vi "GetBin16.vi"(8 "error in (no error)":errorcluster, 11 "MsgPackDeserializer in":refnum<class "MsgPackDeserializer.lvclass">) -> (0 "error out":errorcluster, 2 "data":string, 3 "MsgPackDeserializer out":refnum<class "MsgPackDeserializer.lvclass">)   [LabVIEW 2015, in "MsgPackDeserializer.lvclass"]
uses:
  MsgPackDeserializer.lvclass
  MsgPackDeserializer.lvclass/MsgPackDeserializer.ctl
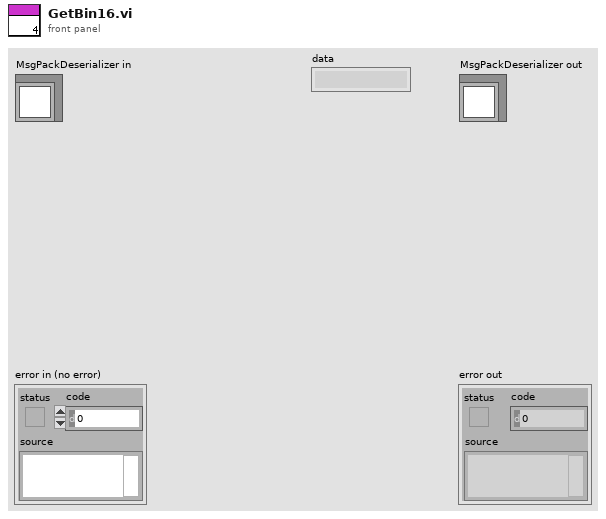
[diagram p1: front panel]
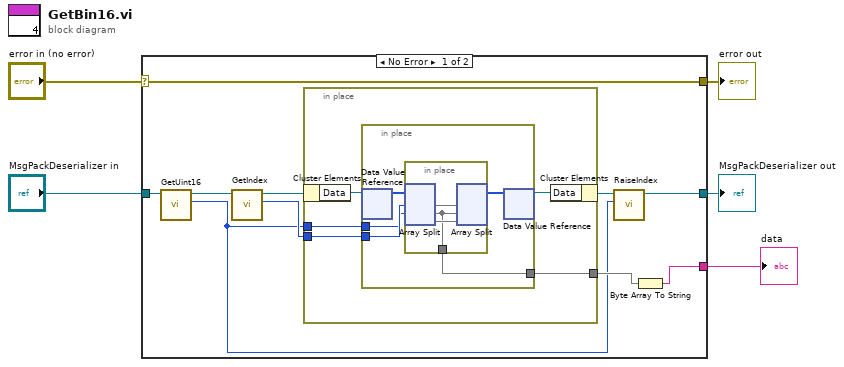
[diagram p0: block diagram]
diagram:
  n1 = case shown="No Error" "error in (no error)" {
    selector: "error in (no error)" -> [w15 w30]
    tunnel: [w15 w30] -> w4
    tunnel: [w7 w29] -> w2
    tunnel: "MsgPackDeserializer in" -> [w11 w29]
    tunnel: [w6 _] -> w1
    frame No Error {
      n2 = call "GetUint16.vi"("MsgPackDeserializer in"=w11) -> ("Number"=w8:u16, "MsgPackDeserializer out"=w10:refnum<class "MsgPackDeserializer.lvclass">)  [unwired: 8 in, 1 out]
      n3 = call "GetIndex.vi"("MsgPackDeserializer in"=w10) -> ("Index"=w12:i64, "MsgPackDeserializer out"=w13:refnum<class "MsgPackDeserializer.lvclass">)  [unwired: 8 in, 1 out]
      n4 = in-place {
        in-place-border: w12 -> [w18]
        in-place-border: w8 -> [w17]
        in-place-border: [w16] -> w9
        n5 = in-place-cluster #1(w13) -> ("Data"=w20:refnum<data-value>)
        n6 = in-place {
          in-place-border: w18 -> [w24]
          in-place-border: w17 -> [w23]
          in-place-border: [w22] -> w16
          n7 = in-place-dvr #2(w20) -> (w25:u8[])  [unwired: 1 out]
          n8 = in-place {
            in-place-border: [w26] -> w22
            n9 = in-place-split #3(w25, w24, w23) -> (w27:u8[], w26:u8[], w28:u8[])
            n10 = in-place-split #3(w27, w26, w28) -> (w21:u8[])  [unwired: 2 out]
          }
          n11 = in-place-dvr #2(w21) -> (w19:refnum<data-value>)  [unwired: 1 out]
        }
        n12 = in-place-cluster #1("Data"=w19) -> (w14:refnum<class "MsgPackDeserializer.lvclass">)
      }
      n13 = call "RaiseIndex.vi"("x"=w8, "MsgPackDeserializer in"=w14) -> ("MsgPackDeserializer out"=w7:refnum<class "MsgPackDeserializer.lvclass">)  [unwired: 8 in, 1 out]
      n14 = Byte Array To String(unsigned byte array=w9) -> (string=w6:string)
    }
    frame Error {
    }
  }
  "error out" <- w4
  "MsgPackDeserializer out" <- w2
  "data" <- w1
